vi "_Waveform.vi"   [LabVIEW 2015]
uses:
  WaveformControllerState.ctl
  <vilib>/DAQmx/write.llb/DAQmx Write (Digital 1D Wfm NChan NSamp).vi
  <vilib>/DAQmx/write.llb/DAQmx Write (Analog 1D Wfm NChan NSamp).vi
  <vilib>/DAQmx/configure/timing.llb/DAQmx Timing (Sample Clock).vi
  <vilib>/Waveform/DWDTOps.llb/DWDT Uncompress Digital.vi
  <vilib>/DAQmx/miscellaneous.llb/DAQmx Fill In Error Info.vi
  <vilib>/DAQmx/create/channels.llb/DAQmx Create Channel (AO-Voltage-Basic).vi
  <vilib>/DAQmx/create/channels.llb/DAQmx Create Channel (DO-Digital Output).vi
types:
  T1 = cluster{"Piezo Position /um":dbl, "Exposure/ms":dbl, "Samples/millisecond":dbl, "Relax/ms":dbl}
  T2 = typedef "WaveformControllerState.ctl" = enum16{"XY", "runWaves", "generateWaves", "deInit", "Init", "Idle"}
  T3 = cluster{T2, cluster{"Piezo Position /um":dbl, "Exposure/ms":dbl, "Samples/millisecond":dbl, "Relax/ms":dbl}}
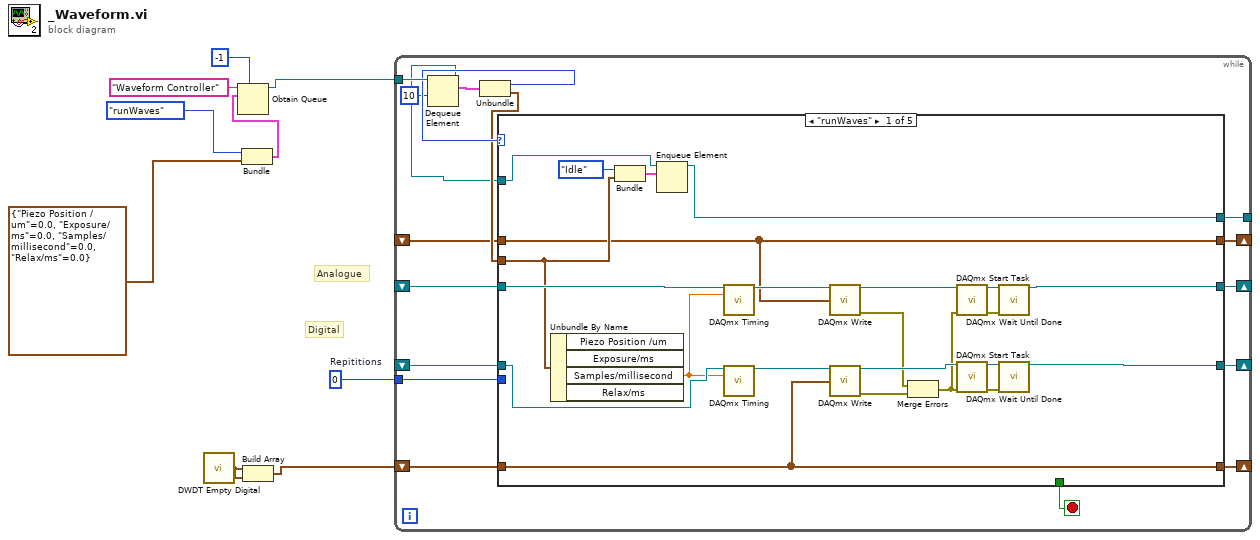
[diagram p0: block diagram]
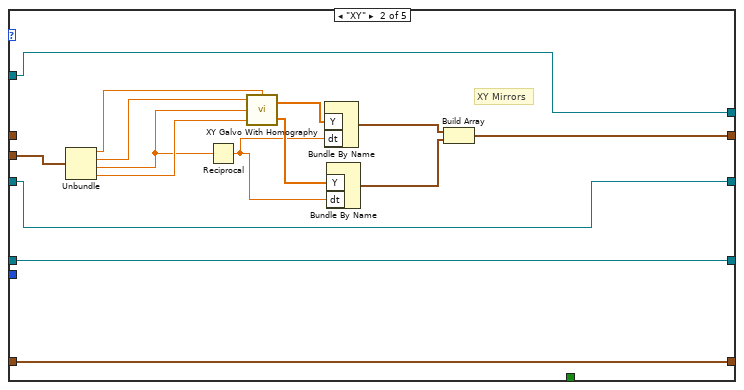
[diagram p2: hidden frame]
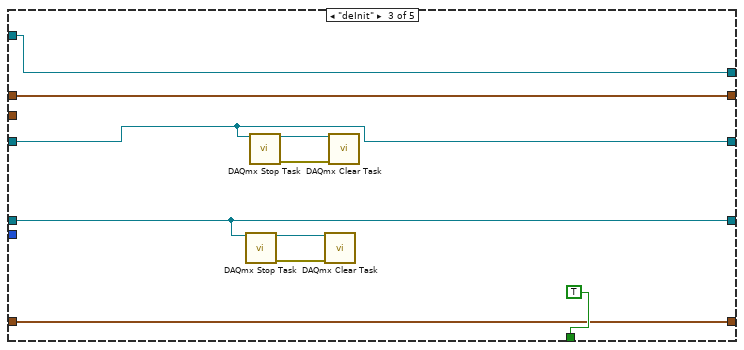
[diagram p3: hidden frame]
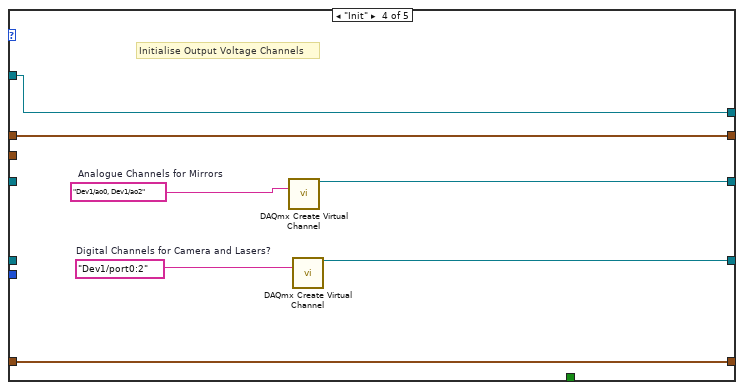
[diagram p4: hidden frame]
diagram:
  w4 = 0  # Repititions
  # "Digital"
  # "Analogue"
  n1 = call <vilib>:"DWDT Empty Digital.vi"() -> ("digital waveform out"=w2:digitalwaveform)  [unwired: 5 in]
  n2 = Bundle(WaveformControllerState."runWaves", T1 {"Piezo Position /um"=0.0, "Exposure/ms"=0.0, "Samples/millisecond"=0.0, "Relax/ms"=0.0}) -> (w5:T3)  [unwired: 1 in]
  n3 = Obtain Queue(max queue size (-1, unlimited)=-1, name (unnamed)="Waveform Controller", element data type=w5) -> (queue out=w8:refnum<queue>)  [unwired: 2 in, 2 out]
  n4 = Build Array(w2, w2) -> (w3:digitalwaveform[])
  n5 = while {
    tunnel: w8 -> [w26]
    shift-right: [w21] -> _
    shift-left: _ -> [w20]
    tunnel: w4 -> [w19]
    tunnel: [w17] -> _
    shift-right: [w15] -> _
    shift-left: _ -> [w13]
    shift-right: [w16] -> _
    shift-left: _ -> [w14]
    shift-right: [w12] -> _
    shift-left: w3 -> [w11]
    stop <- w25 stop-if-true
    n6 = Dequeue Element(queue=w26, timeout in ms (-1)=10) -> (queue out=w18:refnum<queue>, element=w24:T3)  [unwired: 1 in, 2 out]
    n7 = Unbundle(w24) -> (w23:T2, w22:T1)
    n8 = case shown="\"runWaves\"" w23 {
      tunnel: [_ _ TRUE _ _] -> w25
      tunnel: w22 -> [w44 w64 _ _ _]
      tunnel: [w39 w54 w72 w81 w85] -> w21
      tunnel: w20 -> [w39 _ w72 w81 w85]
      tunnel: w19 -> [_ _ _ _ _]
      tunnel: w18 -> [w49 w53 w73 w80 w86]
      tunnel: [w48 w53 w73 w80 w86] -> w17
      tunnel: [w29 w51 w66 w77 w84] -> w16
      tunnel: [w31 w52 w65 w76 w83] -> w15
      tunnel: w14 -> [w43 w51 w66 _ w84]
      tunnel: w13 -> [w45 w52 w65 _ w83]
      tunnel: [w38 w50 w71 w75 w82] -> w12
      tunnel: w11 -> [w38 w50 w71 w75 w82]
      frame "runWaves" {
        n9 = Unbundle By Name(w44) -> ("Samples/millisecond"=w42:dbl)  [unwired: 3 out]
        n10 = Bundle(WaveformControllerState."Idle", w44) -> (w46:T3)  [unwired: 1 in]
        n11 = Enqueue Element(queue=w49, element=w46) -> (queue out=w48:refnum<queue>)  [unwired: 2 in, 2 out]
        n12 = call-poly <vilib>:"DAQmx Timing.vi"("task/channels in"=w45, "rate"=w42) -> ("task out"=w41:refnum<k21>)  [unwired: 12 in, 1 out]
        n13 = call-poly <vilib>:"DAQmx Timing.vi"("task/channels in"=w43, "rate"=w42) -> ("task out"=w40:refnum<k21>)  [unwired: 12 in, 1 out]
        n14 = call-poly <vilib>:"DAQmx Write.vi"("task/channels in"=w41, "data"=w39) -> ("task out"=w37:refnum<k21>, "error out"=w34:errorcluster)  [unwired: 11 in, 1 out]
        n15 = call-poly <vilib>:"DAQmx Write.vi"("task/channels in"=w40, "data"=w38) -> ("task out"=w36:refnum<k21>, "error out"=w35:errorcluster)  [unwired: 11 in, 1 out]
        n16 = Merge Errors(w34, w35) -> (w33:errorcluster)
        n17 = call <vilib>:"DAQmx Start Task.vi"("task/channels in"=w37, "error in"=w33) -> ("task out"=w32:refnum<k21>, "error out"=w27:errorcluster)  [unwired: 12 in]
        n18 = call <vilib>:"DAQmx Start Task.vi"("task/channels in"=w36, "error in"=w33) -> ("task out"=w30:refnum<k21>, "error out"=w28:errorcluster)  [unwired: 12 in]
        n19 = call <vilib>:"DAQmx Wait Until Done.vi"("task/channels in"=w32, "error in"=w27) -> ("task out"=w31:refnum<k21>)  [unwired: 12 in, 1 out]
        n20 = call <vilib>:"DAQmx Wait Until Done.vi"("task/channels in"=w30, "error in"=w28) -> ("task out"=w29:refnum<k21>)  [unwired: 12 in, 1 out]
      }
      frame "XY" {
        # "XY Mirrors"
        n21 = Unbundle(w64) -> ("Piezo Position /um"=w63:dbl, "Exposure/ms"=w62:dbl, "Samples/millisecond"=w59:dbl, "Relax/ms"=w61:dbl)
        n22 = Reciprocal(x=w59) -> (1/x=w57:dbl)
        n23 = call "XY Galvo With Homography.vi"("Piezo Position (um)"=w63, "Relax (ms)"=w61, "Samples /Millisecond"=w59, "Exposure (ms)"=w62) -> ("Z Mirror Signal"=w58:dbl[], "Scan Mirror Signal"=w60:dbl[])
        n24 = Bundle By Name("Y"=w60, "dt"=w57) -> (w55:waveform(dbl))  [unwired: 1 in]
        n25 = Bundle By Name("Y"=w58, "dt"=w57) -> (w56:waveform(dbl))  [unwired: 1 in]
        n26 = Build Array(w55, w56) -> (w54:waveform(dbl)[])
      }
      frame "deInit" {
        n27 = call <vilib>:"DAQmx Stop Task.vi"("task/channels in"=w66) -> ("task out"=w67:refnum<k21>, "error out"=w68:errorcluster)  [unwired: 13 in]
        n28 = call <vilib>:"DAQmx Stop Task.vi"("task/channels in"=w65) -> ("task out"=w70:refnum<k21>, "error out"=w69:errorcluster)  [unwired: 13 in]
        n29 = call <vilib>:"DAQmx Clear Task.vi"("task in"=w67, "error in"=w68) -> ()  [unwired: 13 in, 1 out]
        n30 = call <vilib>:"DAQmx Clear Task.vi"("task in"=w70, "error in"=w69) -> ()  [unwired: 13 in, 1 out]
      }
      frame "Init" {
        w78 = tag "Dev1/port0:2"  # Digital Channels for Camera and Lasers?
        w79 = tag "Dev1/ao0, Dev1/ao2"  # Analogue Channels for Mirrors
        # "Initialise Output Voltage Channels"
        n31 = call-poly <vilib>:"DAQmx Create Virtual Channel.vi"("physical channels"=w79) -> ("task out"=w76:refnum<k21>)  [unwired: 13 in, 1 out]
        n32 = call-poly <vilib>:"DAQmx Create Virtual Channel.vi"("lines"=w78) -> ("task out"=w77:refnum<k21>)  [unwired: 13 in, 1 out]
      }
      frame "Idle", Default {
      }
    }
  }
